vi "Display Title.vi"(8 "error in (no error)":errorcluster, 9 "title":string, 11 "VISA resource name":refnum<visa-resource-name>) -> (0 "error out":errorcluster, 3 "VISA resource name out":refnum<visa-resource-name>)   [LabVIEW 2018, in "Agilent 87XX Series.lvlib"]
doc: "This VI for the HP8753B Network Analyzer is used to write a title to the screen. It is the same as the \"TITLE\" softkey associated with the \"DISPLAY\" button. The title can only be 50 characters.The softkeys on the HP8753B like \"NEWLINE\" and \"LIMIT TEST RESULT\" must be entered as characters like other characters in the title:\n\n NEWLINE - [NL]\n FORMFEED - [FF]\n ACTIVE ENTRY - [ACT]\n ACTIVE MARKER MAGNITUDE - [MKR]\n LIMIT TEST RESULT - [LIMIT]\n LOOP COUNTER - [LOOP]\n END OF LABEL - [EOL]\n\n For longer text only titles, use the \"write text to screen\" VI."
uses:
  Agilent 87XX Series.lvlib
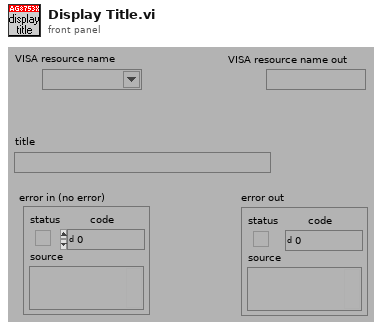
[diagram p1: front panel]
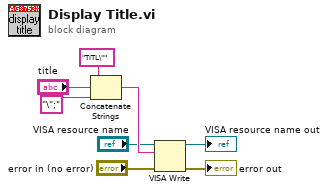
[diagram p0: block diagram]
diagram:
  n1 = Concatenate Strings("TITL\"", "title", "\";") -> (w5:string)
  n2 = VISA Write(VISA resource name="VISA resource name", write buffer=w5, error in (no error)="error in (no error)") -> (VISA resource name out=→"VISA resource name out":refnum<visa-resource-name>, error out=→"error out":errorcluster)  [unwired: 1 out]
